vi "RT_Gravitational_Force_in_DLR_Navigation_Reference_System(SubVI).vi"(0 "Data":dbl[][](array[numeric]), 5 "i":i32, 9 "latd (rad)":dbl format="%#_13g", 11 "alt (m)":dbl format="%#_13g") -> (4 "FG_d":dbl[](array[numeric]), 15 "L_C (rad)":dbl)   [LabVIEW 2011]
panel:
  out "M":dbl
  out "gl_tC":dbl
  out "gl_rC":dbl
  out "R_l (m)":dbl
  out "D_l":dbl
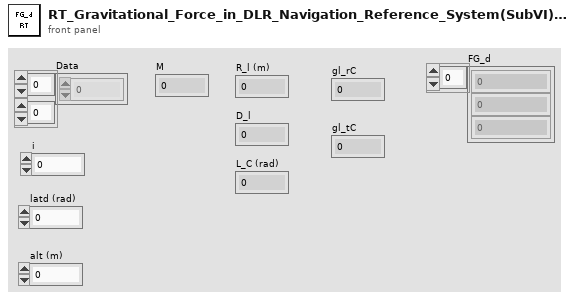
[diagram p1: front panel]
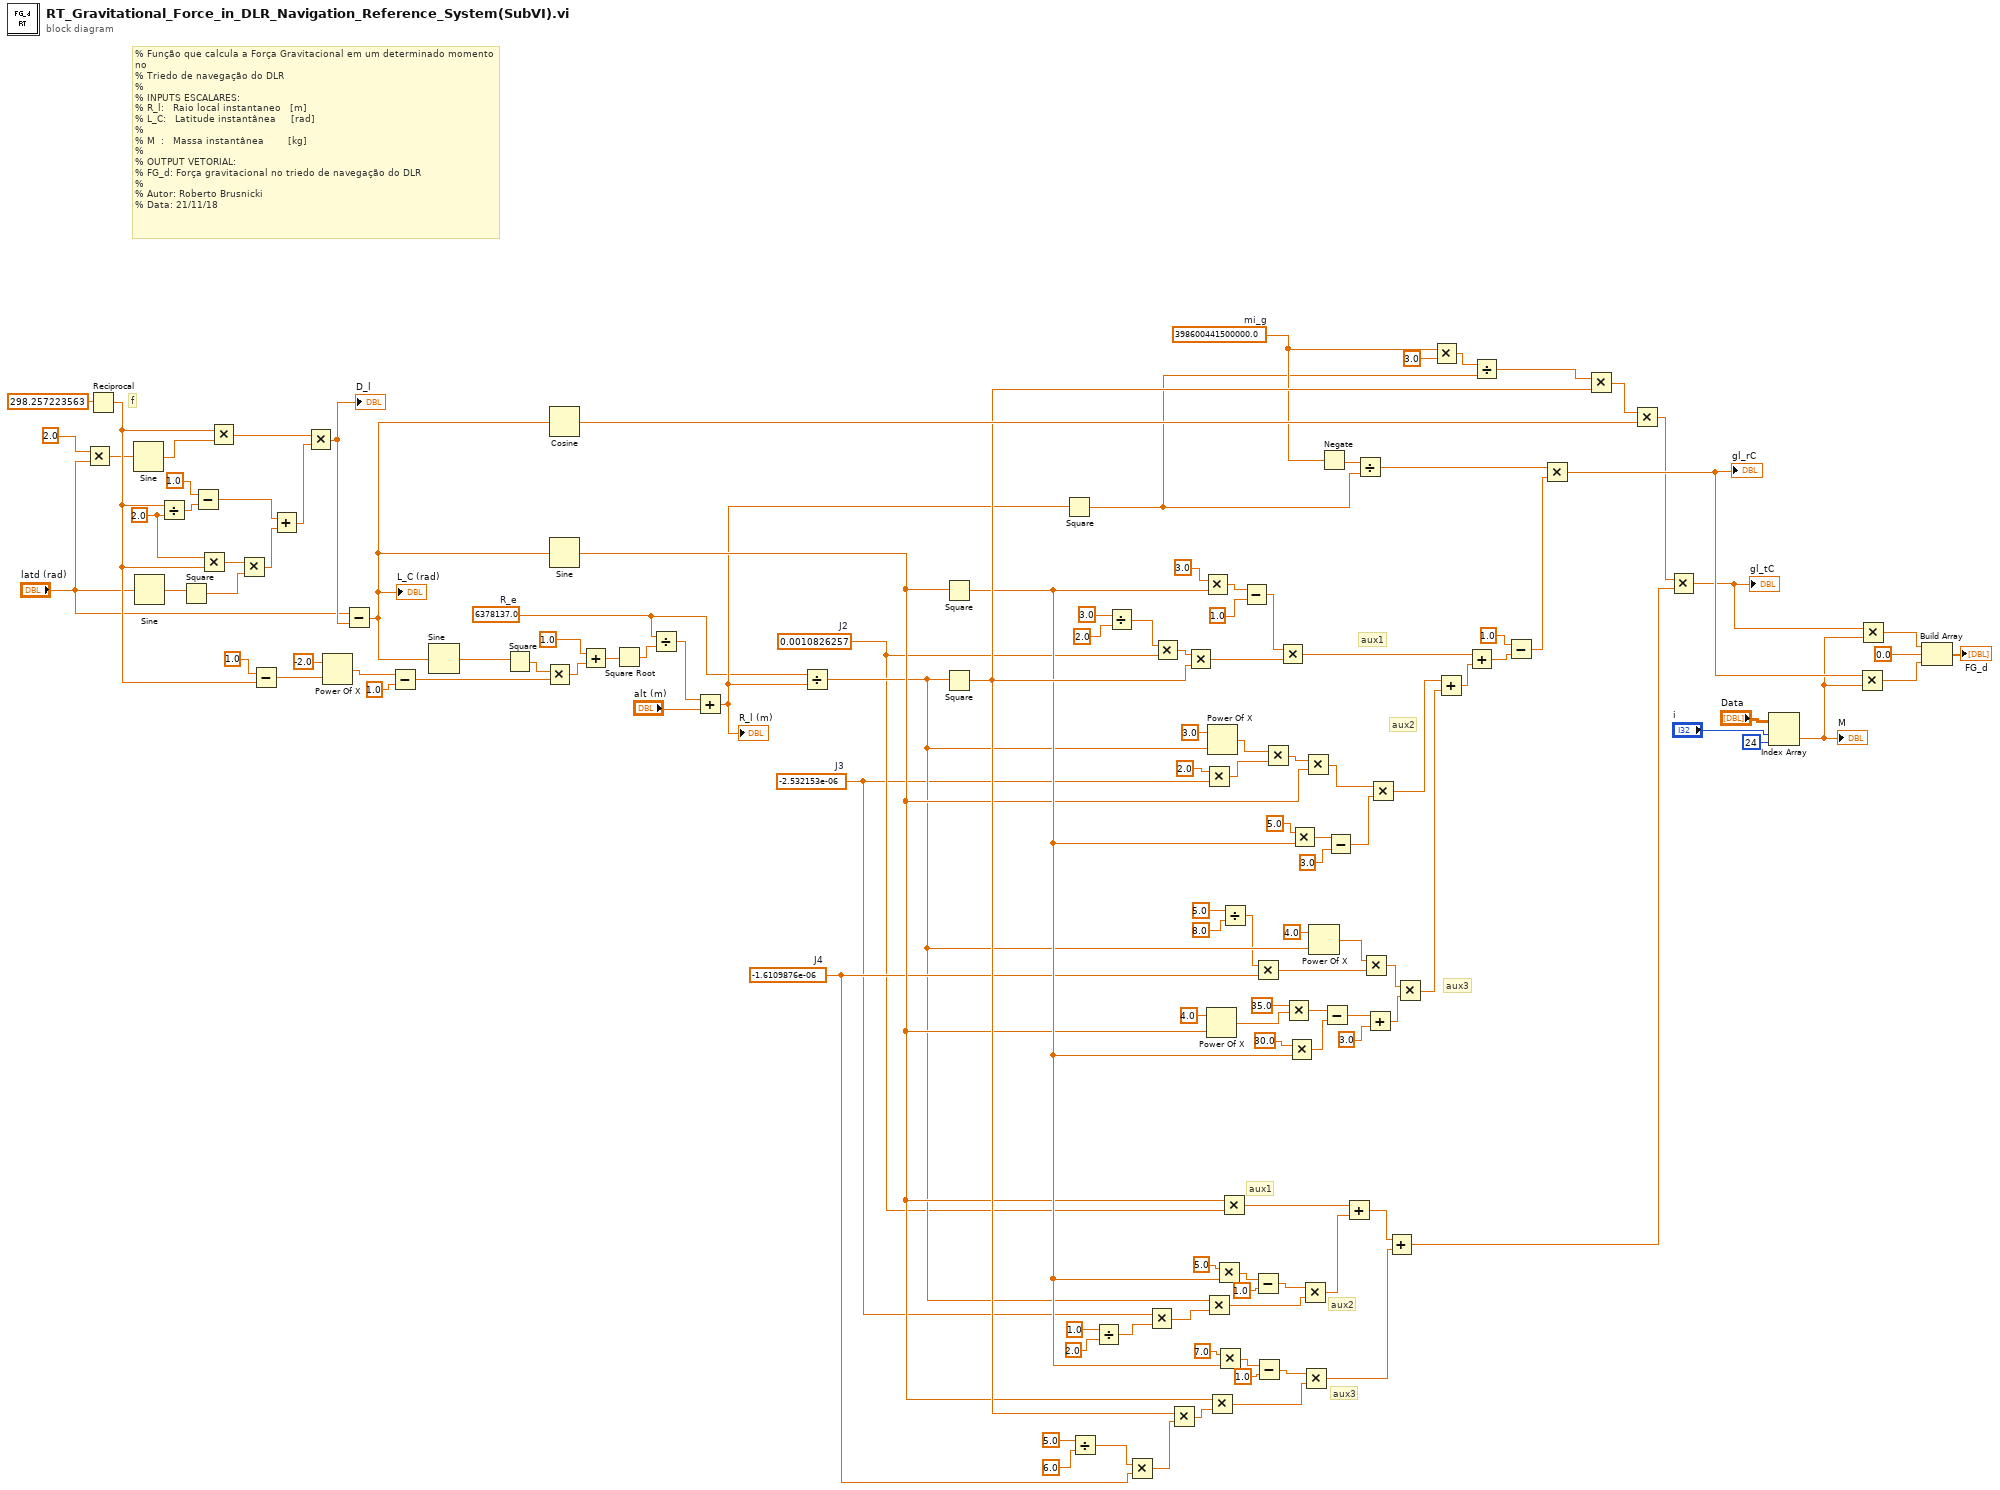
[diagram p0: block diagram]
diagram:
  w93 = -1.6109876e-06  # J4
  w8 = -2.532153e-06  # J3
  w82 = 0.0010826257  # J2
  w104 = 398600441500000.0  # mi_g
  w12 = 2.0 ("y")
  w45 = 6378137.0  # R_e
  # "f"
  # "aux3"
  # "aux2"
  # "aux1"
  # "aux3"
  # "aux2"
  # "aux1"
  # "% Função que calcula a Força Gravitacional em um determinado momento no \n% Triedo de navegação do DLR\n%\n% INPUTS ESCALARES: \n% R_l:   Raio local instantaneo   [m]\n% L_C:   Latitude instantânea     [rad]\n% \n% M  :   Massa instantânea        [kg]\n%\n% OUTPUT VETORIAL:\n% FG_d: Força gravitacional no triedo de navegação do DLR\n%\n% Autor: Roberto Brusnicki\n% Data: 21/11/18"
  n1 = Multiply(x=2.0, y="latd (rad)") -> (x*y=w15:dbl)
  n2 = Reciprocal(x=298.257223563) -> (1/x=w29:dbl)
  n3 = Sine(x=w15) -> (sin(x)=w16:dbl)
  n4 = Sine(x="latd (rad)") -> (sin(x)=w20:dbl)
  n5 = Divide(x=w29, y=w12) -> (x/y=w18:dbl)
  n6 = Square(x=w20) -> (x^2=w22:dbl)
  n7 = Subtract(x=1.0, y=w18) -> (x-y=w23:dbl)
  n8 = Multiply(x=w12, y=w29) -> (x*y=w21:dbl)
  n9 = Multiply(x=w29, y=w16) -> (x*y=w17:dbl)
  n10 = Multiply(x=w21, y=w22) -> (x*y=w24:dbl)
  n11 = Subtract(x=1.0, y=w29) -> (x-y=w30:dbl)
  n12 = Add(x=w23, y=w24) -> (x+y=w25:dbl)
  n13 = Multiply(x=w17, y=w25) -> (x*y=w27:dbl)
  "D_l" <- w27
  n14 = Power Of X(1:w30, 2:-2.0 ("y")) -> (0:w32:dbl)
  n15 = Subtract(x="latd (rad)", y=w27) -> (x-y=w111:dbl)
  "L_C (rad)" <- w111
  n16 = Subtract(x=w32, y=1.0) -> (x-y=w37:dbl)
  n17 = Sine(x=w111) -> (sin(x)=w35:dbl)
  n18 = Square(x=w35) -> (x^2=w36:dbl)
  n19 = Multiply(x=w36, y=w37) -> (x*y=w38:dbl)
  n20 = Cosine(x=w111) -> (cos(x)=w110:dbl)
  n21 = Sine(x=w111) -> (sin(x)=w96:dbl)
  n22 = Add(x=1.0, y=w38) -> (x+y=w39:dbl)
  n23 = Square Root(x=w39) -> (sqrt(x)=w40:dbl)
  n24 = Divide(x=w45, y=w40) -> (x/y=w41:dbl)
  n25 = Add(x=w41, y="alt (m)") -> (x+y=w74:dbl)
  "R_l (m)" <- w74
  n26 = Divide(x=w45, y=w74) -> (x/y=w83:dbl)
  n27 = Square(x=w96) -> (x^2=w101:dbl)
  n28 = Square(x=w83) -> (x^2=w107:dbl)
  n29 = Square(x=w74) -> (x^2=w103:dbl)
  n30 = Divide(x=5.0, y=6.0 ("x")) -> (x/y=w90:dbl)
  n31 = Divide(x=1.0, y=2.0) -> (x/y=w10:dbl)
  n32 = Divide(x=3.0, y=2.0) -> (x/y=w44:dbl)
  n33 = Multiply(x=w90, y=w93) -> (x*y=w94:dbl)
  n34 = Multiply(x=w8, y=w10) -> (x*y=w9:dbl)
  n35 = Multiply(x=w44, y=w82) -> (x*y=w46:dbl)
  n36 = Multiply(x=w107, y=w94) -> (x*y=w95:dbl)
  n37 = Multiply(x=w46, y=w107) -> (x*y=w47:dbl)
  n38 = Multiply(x=3.0, y=w101) -> (x*y=w49:dbl)
  n39 = Multiply(x=2.0, y=w8) -> (x*y=w55:dbl)
  n40 = Multiply(x=w83, y=w9) -> (x*y=w11:dbl)
  n41 = Power Of X(1:w96, 2:4.0 ("y")) -> (0:w68:dbl)
  n42 = Power Of X(1:w83, 2:3.0 ("y")) -> (0:w54:dbl)
  n43 = Multiply(x=w96, y=w95) -> (x*y=w102:dbl)
  n44 = Multiply(x=5.0, y=w101) -> (x*y=w87:dbl)
  n45 = Multiply(x=7.0, y=w101) -> (x*y=w99:dbl)
  n46 = Multiply(x=w96, y=w82) -> (x*y=w112:dbl)
  n47 = Divide(x=5.0, y=8.0 ("x")) -> (x/y=w62:dbl)
  n48 = Subtract(x=w49, y=1.0) -> (x-y=w51:dbl)
  n49 = Multiply(x=w62, y=w93) -> (x*y=w65:dbl)
  n50 = Subtract(x=w87, y=1.0) -> (x-y=w89:dbl)
  n51 = Subtract(x=w99, y=1.0) -> (x-y=w97:dbl)
  n52 = Multiply(x=w54, y=w55) -> (x*y=w56:dbl)
  n53 = Multiply(x=w51, y=w47) -> (x*y=w77:dbl)
  n54 = Multiply(x=35.0, y=w68) -> (x*y=w69:dbl)
  n55 = Multiply(x=30.0, y=w101) -> (x*y=w3:dbl)
  n56 = Multiply(x=5.0, y=w101) -> (x*y=w6:dbl)
  n57 = Multiply(x=w89, y=w11) -> (x*y=w113:dbl)
  n58 = Multiply(x=w97, y=w102) -> (x*y=w115:dbl)
  n59 = Multiply(x=w56, y=w96) -> (x*y=w57:dbl)
  n60 = Power Of X(1:w83, 2:4.0 ("y")) -> (0:w64:dbl)
  n61 = Negate(x=w104) -> (-x=w73:dbl)
  n62 = Subtract(x=w69, y=w3) -> (x-y=w2:dbl)
  n63 = Subtract(x=w6, y=3.0) -> (x-y=w5:dbl)
  n64 = Add(x=w112, y=w113) -> (x+y=w114:dbl)
  n65 = Divide(x=w73, y=w103) -> (x/y=w80:dbl)
  n66 = Multiply(x=w64, y=w65) -> (x*y=w72:dbl)
  n67 = Add(x=w2, y=3.0) -> (x+y=w1:dbl)
  n68 = Multiply(x=w57, y=w5) -> (x*y=w4:dbl)
  n69 = Add(x=w114, y=w115) -> (x+y=w117:dbl)
  n70 = Multiply(x=w72, y=w1) -> (x*y=w78:dbl)
  n71 = Multiply(x=w104, y=3.0) -> (x*y=w106:dbl)
  n72 = Add(x=w4, y=w78) -> (x+y=w79:dbl)
  n73 = Add(x=w77, y=w79) -> (x+y=w76:dbl)
  n74 = Divide(x=w106, y=w103) -> (x/y=w108:dbl)
  n75 = Subtract(x=1.0, y=w76) -> (x-y=w81:dbl)
  n76 = Multiply(x=w80, y=w81) -> (x*y=w125:dbl)
  "gl_rC" <- w125
  n77 = Multiply(x=w108, y=w107) -> (x*y=w109:dbl)
  n78 = Multiply(x=w109, y=w110) -> (x*y=w116:dbl)
  n79 = Multiply(x=w116, y=w117) -> (x*y=w123:dbl)
  "gl_tC" <- w123
  n80 = Index Array(array="Data", index (row)="i", index (col)=24 ("disabled index (col)")) -> (element=w122:dbl)
  "M" <- w122
  n81 = Multiply(x=w125, y=w122) -> (x*y=w126:dbl)
  n82 = Multiply(x=w123, y=w122) -> (x*y=w124:dbl)
  n83 = Build Array(w124, 0.0 ("y"), w126) -> (→"FG_d":dbl[])
